vi "MotionControl_API_Test.vi"() -> ()   [LabVIEW 2010]
uses:
  labbCAN_Bus_API/labbCAN_Bus_API.lvlib
  labbCAN_MotionControl_API/labbCAN_MotionControl_API.lvlib
panel:
  out "TargetPosReached":bool
  out "Position Y":dbl
  out "Position X":dbl
  out "Axis Homing Attained":bool
  out "error out":errorcluster caption="Fehler (Ausgang)"
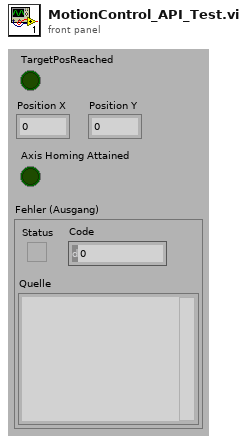
[diagram p1: front panel]
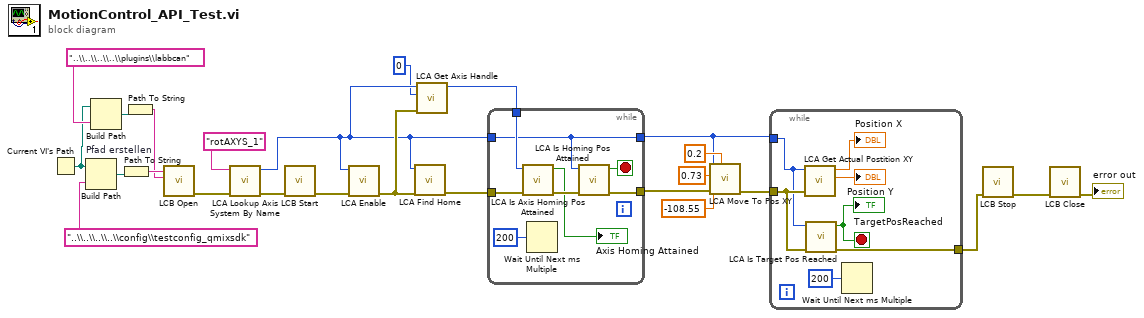
[diagram p0: block diagram]
diagram:
  n1 = Current VI's Path() -> (path=w2:path)
  n2 = Build Path "Pfad erstellen"(base path=w2, name or relative path="..\\..\\..\\..\\config\\testconfig_qmixsdk" ("Name oder relativer Pfad")) -> (appended path=w5:path)
  n3 = Build Path(base path=w2, name or relative path="..\\..\\..\\..\\plugins\\labbcan" ("Name oder relativer Pfad")) -> (appended path=w4:path)
  n4 = Path To String(path=w5) -> (string=w24:string)
  n5 = Path To String(path=w4) -> (string=w1:string)
  n6 = call "LCB Open.vi"("PluginSearchPath"=w1, "Device Configuration Path"=w24) -> ("error out"=w23:errorcluster)  [unwired: 9 in]
  n7 = call "LCA Lookup Axis System By Name.vi"("error in (no error)"=w23, "Axis System Name"="rotAXYS_1" ("pAxisName")) -> ("error out"=w21:errorcluster, "Axis System Handle"=w16:i64)  [unwired: 8 in]
  n8 = call "LCB Start.vi"("error in (no error)"=w21) -> ("error out"=w19:errorcluster)  [unwired: 10 in]
  n9 = call "LCA Enable.vi"("error in (no error)"=w19, "Axis System Handle"=w16) -> ("error out"=w17:errorcluster)  [unwired: 9 in]
  n10 = call "LCA Find Home.vi"("error in (no error)"=w17, "Axis System Handle"=w16) -> ("error out"=w18:errorcluster)  [unwired: 9 in]
  n11 = call "LCA Get Axis Handle.vi"("error in (no error)"=w17, "Axis Index"=u8 0 ("AxisId"), "Axis System Handle"=w16) -> ("AxisHandle"=w14:i64)  [unwired: 7 in, 1 out]
  n12 = while {
    tunnel: w18 -> [w30]
    tunnel: w16 -> [w26]
    tunnel: [w32] -> w13
    tunnel: w14 -> [w28]
    tunnel: [w26] -> w8
    stop <- w33 stop-if-true
    n13 = call "LCA Is Axis Homing Pos Attained.vi"("error in (no error)"=w30, "Axis Handle"=w28) -> ("error out"=w29:errorcluster, "Homing Attained"=→"Axis Homing Attained":bool)  [unwired: 8 in]
    n14 = Wait Until Next ms Multiple(millisecond multiple=u32 200 ("Vielfache von ms")) -> ()  [unwired: 1 out]
    n15 = call "LCA Is Homing Pos Attained.vi"("error in (no error)"=w29, "Axis System Handle"=w26) -> ("error out"=w32:errorcluster, "Homing Attained"=w33:bool)  [unwired: 8 in]
  }
  n16 = call "LCA Move To Pos XY.vi"("Velocity"=0.2 ("fVelocity"), "error in (no error)"=w13, "Position Y"=-108.55 ("fPositionY"), "Position X"=0.73 ("fPositionX"), "Axis System Handle"=w8) -> ("error out"=w9:errorcluster)  [unwired: 6 in]
  n17 = while {
    tunnel: w9 -> [w38]
    tunnel: w8 -> [w37]
    tunnel: [w36] -> w7
    stop <- w34 stop-if-true
    n18 = call "LCA Get Actual Postition XY.vi"("error in (no error)"=w38, "Axis System Handle"=w37) -> ("Position Y"=→"Position Y":dbl, "Position X"=→"Position X":dbl)  [unwired: 7 in, 1 out]
    n19 = call "LCA Is Target Pos Reached.vi"("error in (no error)"=w38, "Axis System Handle"=w37) -> ("error out"=w36:errorcluster, "Target Reached"=w34:bool)  [unwired: 8 in]
    "TargetPosReached" <- w34
    n20 = Wait Until Next ms Multiple(millisecond multiple=u32 200 ("Vielfache von ms")) -> ()  [unwired: 1 out]
  }
  n21 = call "LCB Stop.vi"("error in (no error)"=w7) -> ("error out"=w20:errorcluster)  [unwired: 10 in]
  n22 = call "LCB Close.vi"("error in (no error)"=w20) -> ("error out"=→"error out":errorcluster)  [unwired: 10 in]
